vi "Get Channel Info.vi"(8 "error in":errorcluster, 11 "refnum in":refnum<file>) -> (0 "error out":errorcluster, 1 "time":dbl format="%.2f", 2 "channel information":T1(array[cluster]) {"sensor sensitivity (mV/EU)" format="%.2f"; "offset" format="%.2f"; "multiplier" format="%.2f"}, 3 "dup refnum":refnum<file>, 4 "data offset":i32, 5 "Sample rate":sgl format="%.2f")   [LabVIEW 2017]
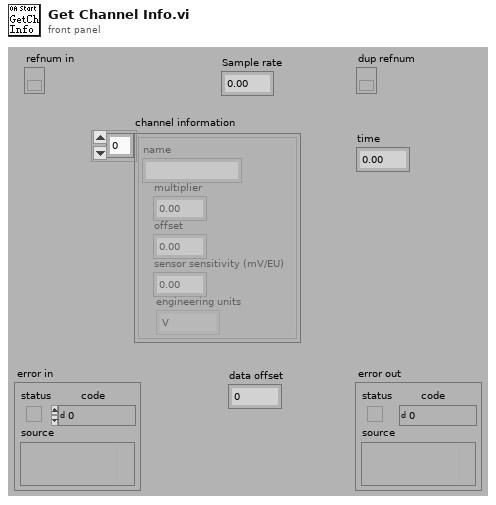
[diagram p1: front panel]
types:
  T1 = cluster{"name":string, "multiplier":sgl, "offset":sgl, "sensor sensitivity (mV/EU)":dbl, "engineering units":enum16{"custom...", "V", "Pa", "g", "m/s^2", "m/s", "m", "in/s^2", "in/s", "in"}}[]
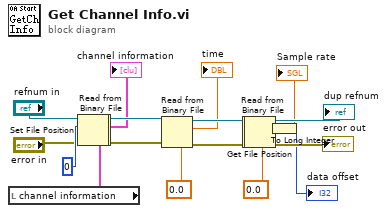
[diagram p0: block diagram]
diagram:
  n1 = local read "channel information"() -> (w9:T1)
  n2 = Set File Position(offset (in bytes) (0)=0 ("pos offset (0)"), refnum="refnum in", error in="error in") -> (refnum out=w2:refnum<file>, error out=w1:errorcluster)  [unwired: 1 in]
  n3 = Read from Binary File(5:w9, 8:w1, 11:w2) -> (0:w19:errorcluster, 2:→"channel information":T1, 3:w21:refnum<file>)  [unwired: 3 in, 1 out]
  n4 = Read from Binary File(5:0.0 ("Sample rate"), 8:w19, 11:w21) -> (0:w16:errorcluster, 2:→"time":dbl, 3:w18:refnum<file>)  [unwired: 3 in, 1 out]
  n5 = Read from Binary File(5:sgl 0.0 ("Sample rate"), 8:w16, 11:w18) -> (0:w4:errorcluster, 2:→"Sample rate":sgl, 3:w5:refnum<file>)  [unwired: 3 in, 1 out]
  n6 = Get File Position(4:w4, 7:w5) -> (0:→"error out":errorcluster, 2:w3:i64, 3:→"dup refnum":refnum<file>)
  n7 = To Long Integer(number=w3) -> (32bit integer=→"data offset":i32)
